vi "SOAE-Process Sample.vi"(0 "runtime in":T1, 1 "Graph":refnum<vi>) -> (4 "runtime out":T1, 8 "finished":bool, 14 "acquired":i32, 15 "error out":errorcluster)   [LabVIEW 2020]
uses:
  Typedefs/SOAE-Acq Runtime.ctl
  <vilib>/DAQmx/read.llb/DAQmx Read (Analog 1D DBL 1Chan NSamp).vi
  <vilib>/DAQmx/miscellaneous.llb/DAQmx Fill In Error Info.vi
  Utility VIs/Math VIs/FFT x(t) to dB,Degrees (1D).vi
  Utility VIs/Math VIs/dB to Linear (1D).vi
  Utility VIs/Math VIs/Linear to dB (array).vi
  <vilib>/Analysis/3filter.llb/FIR Filter (DBL).vi
  <vilib>/Analysis/NI_AALBase.lvlib
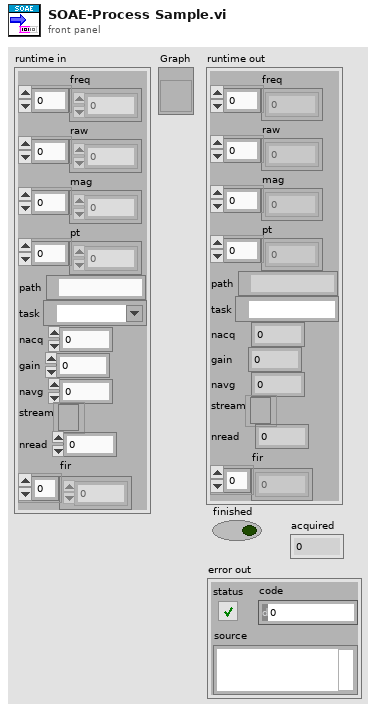
[diagram p1: front panel]
types:
  T1 = typedef "SOAE-Acq Runtime.ctl" = cluster{"freq":dbl[], "raw":dbl[], "mag":dbl[], "pt":dbl[], "path":path, "task":refnum<k21>, "nacq":i32, "gain":dbl, "navg":i32, "stream":refnum<file>, "nread":i32, "fir":dbl[]}
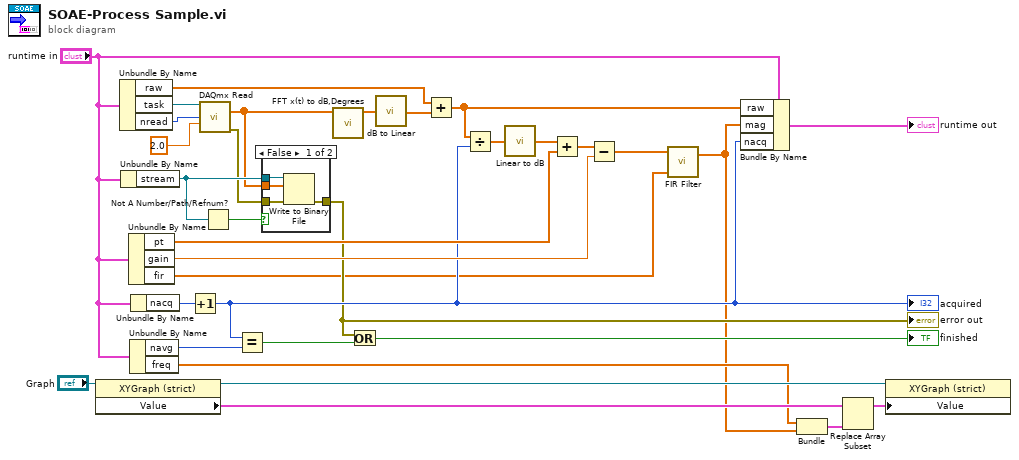
[diagram p0: block diagram]
diagram:
  n1 = property class="XYGraph (strict)"(reference="Graph") -> (reference out=w16:refnum<vi>, "Value"=w15:cluster{"X":dbl[], "Y":dbl[]}[])  [unwired: 1 in, 1 out]
  n2 = Unbundle By Name("runtime in") -> ("raw"=w30:dbl[], "task"=w33:refnum<k21>, "nread"=w5:i32)
  n3 = Unbundle By Name("runtime in") -> ("stream"=w12:refnum<file>)
  n4 = Unbundle By Name("runtime in") -> ("pt"=w25:dbl[], "gain"=w23:dbl, "fir"=w1:dbl[])
  n5 = Unbundle By Name("runtime in") -> ("navg"=w20:i32, "freq"=w8:dbl[])
  n6 = Unbundle By Name("runtime in") -> ("nacq"=w29:i32)
  n7 = Increment(x=w29) -> (x+1=w21:i32)
  "acquired" <- w21
  n8 = call-poly <vilib>:"DAQmx Read.vi"("task/channels in"=w33, "number of samples per channel"=w5, "timeout"=2.0) -> ("data"=w11:dbl[], "error out"=w10:errorcluster)  [unwired: 10 in, 1 out]
  n9 = Not A Number/Path/Refnum?(number/path/refnum=w12) -> (NaN/Path/Refnum?=w13:bool)
  n10 = Equal?(x=w21, y=w20) -> (x = y?=w19:bool)
  n11 = case shown="False" w13 {
    tunnel: w12 -> [w37 _]
    tunnel: w11 -> [w36 _]
    tunnel: [w35 w38] -> w9
    tunnel: w10 -> [w34 w38]
    frame False {
      n12 = Write to Binary File(file (use dialog)=w37, data=w36, error in=w34) -> (error out=w35:errorcluster)  [unwired: 3 in, 2 out]
    }
    frame True {
    }
  }
  "error out" <- w9
  n13 = call-poly "FFT x(t) to dB,Degrees.vi"("X"=w11) -> ("+Freq. Mag of FFT (dB rms)"=w31:dbl[])  [unwired: 8 in, 2 out]
  n14 = Or(x=w9, y=w19) -> (x .or. y?=→"finished":bool)
  n15 = call-poly "dB to Linear.vi"("dB"=w31) -> ("linear"=w6:dbl[])
  n16 = Add(x=w30, y=w6) -> (x+y=w28:dbl[])
  n17 = Divide(x=w28, y=w21) -> (x/y=w27:dbl[])
  n18 = call-poly "Linear to dB.vi"("linear"=w27) -> ("dB"=w26:dbl[])
  n19 = Add(x=w26, y=w25) -> (x+y=w24:dbl[])
  n20 = Subtract(x=w24, y=w23) -> (x-y=w3:dbl[])
  n21 = call-poly <vilib>:"FIR Filter.vi"("FIR Coefficients"=w1, "X"=w3) -> ("Filtered X"=w2:dbl[])  [unwired: 2 in, 1 out]
  n22 = Bundle By Name(cluster="runtime in", "raw"=w28, "mag"=w2, "nacq"=w21) -> (→"runtime out":T1)
  n23 = Bundle("freq"=w8, "Filtered X"=w2) -> (w7:cluster{"freq":dbl[], "Filtered X":dbl[]})  [unwired: 1 in]
  n24 = Replace Array Subset(array=w15, new element=w7) -> (w4:cluster{"X":dbl[], "Y":dbl[]}[])  [unwired: 1 in]
  n25 = property class="XYGraph (strict)"(reference=w16, "Value"=w4) -> ()  [unwired: 1 in, 2 out]
